vi "Write MERCANCÍA.vi"(8 "error in (no error)":errorcluster, 10 "MERCANCÍA":refnum<vi>, 11 "BD_CAFÉ_USD_ESP in":refnum<class "BD_CAFÉ_USD_ESP.lvclass">) -> (0 "error out":errorcluster, 3 "BD_CAFÉ_USD_ESP out":refnum<class "BD_CAFÉ_USD_ESP.lvclass">)   [LabVIEW 2019, in "BD_CAFÉ_USD_ESP.lvlib" / "BD_CAFÉ_USD_ESP.lvclass"]
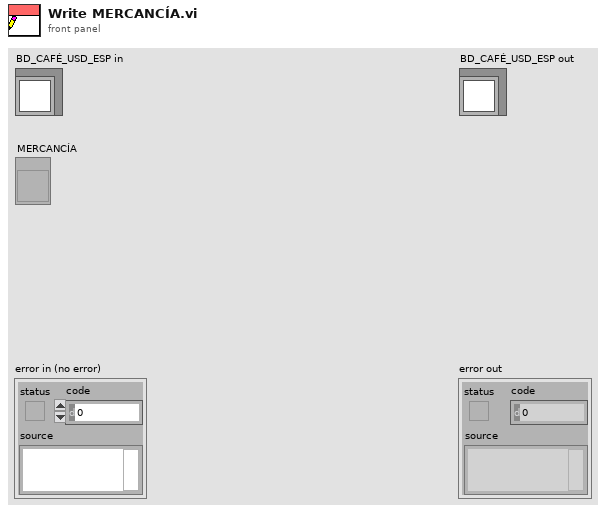
[diagram p1: front panel]
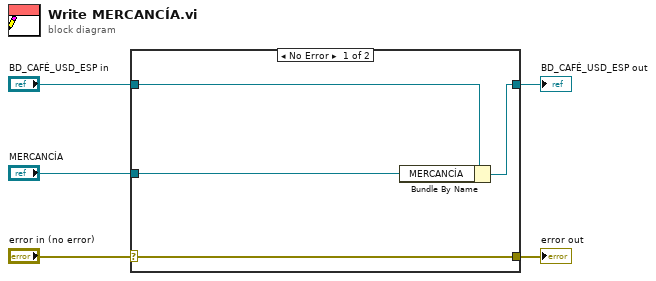
[diagram p0: block diagram]
diagram:
  n1 = case shown="No Error" "error in (no error)" {
    selector: "error in (no error)" -> [w9 w10]
    tunnel: [w9 w10] -> w4
    tunnel: [w7 w11] -> w2
    tunnel: "BD_CAFÉ_USD_ESP in" -> [w8 w11]
    tunnel: "MERCANCÍA" -> [w6 _]
    frame No Error {
      n2 = Bundle By Name(cluster=w8, "MERCANCÍA"=w6) -> (w7:refnum<class "BD_CAFÉ_USD_ESP.lvclass">)
    }
    frame Error {
    }
  }
  "error out" <- w4
  "BD_CAFÉ_USD_ESP out" <- w2
